vi "excavator1D_array.vi"(0 "Name":string, 1 "Array":dbl[][](array[numeric]) format="%#_13g", 2 "x_max":dbl, 3 "x_min":dbl, 4 "Save?":bool) -> (5 "xPoints":i32=263)   [LabVIEW 2013]
panel:
  in  "Tab Control":enum32{"Page 1", "Page 2"}(tab)
  in  "Ring":u16(ring)=1 items=["Windows", "Mac"]
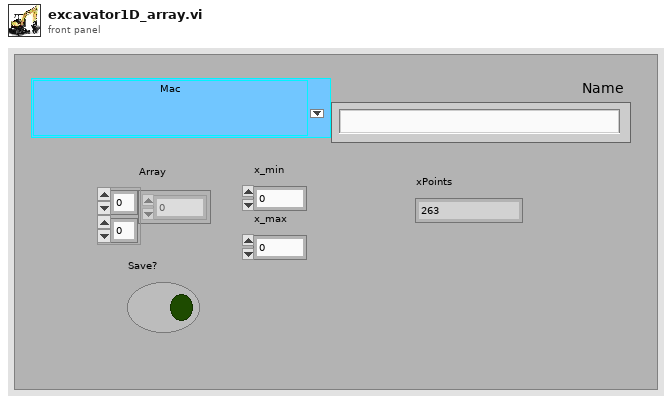
[diagram p1: front panel]
types:
  T1 = enum16{"open", "replace", "create", "open or create", "replace or create", "replace or create with confirmation"}
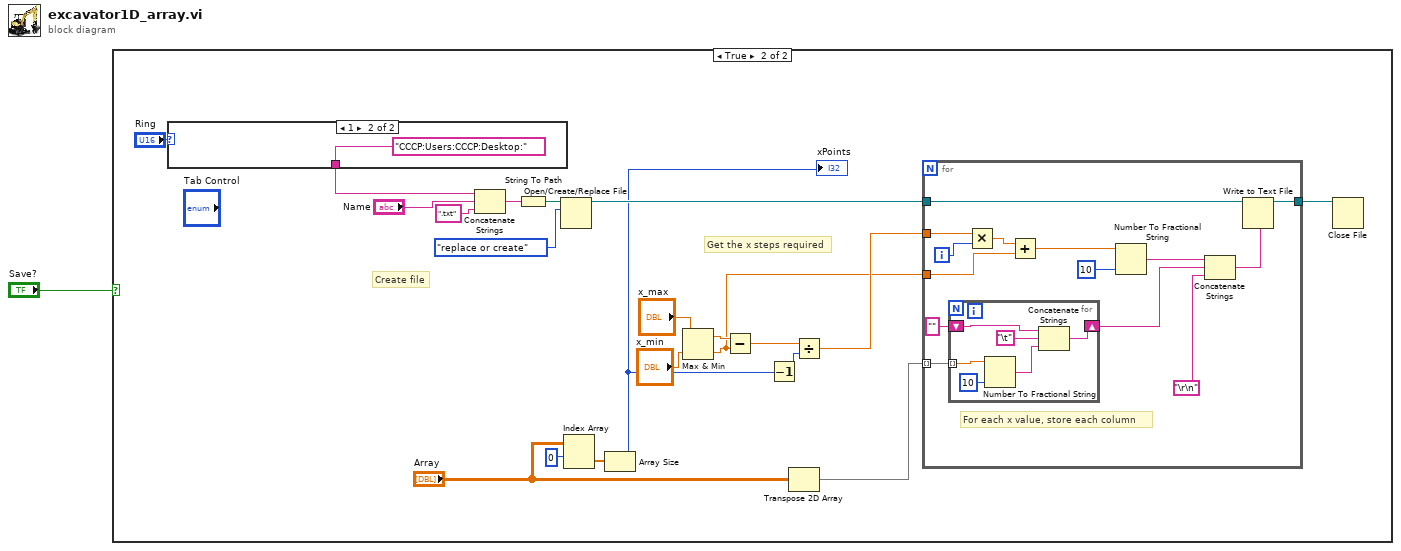
[diagram p0: block diagram]
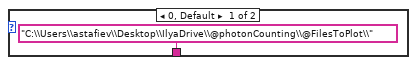
[diagram p3: hidden frame]
diagram:
  n1 = case shown="True" "Save?" {
    frame False {
    }
    frame True {
      # "Create file"
      # "Get the x steps required"
      n2 = case shown="1" "Ring" {
        tunnel: ["C:\\Users\\astafiev\\Desktop\\IlyaDrive\\@photonCounting\\@FilesToPlot\\" ("Directory") "CCCP:Users:CCCP:Desktop:" ("Directory")] -> w11
        frame 0, Default {
        }
        frame 1 {
        }
      }
      n3 = Concatenate Strings(w11, "Name", ".txt" ("FileName 2")) -> (w22:string)
      n4 = String To Path(string=w22) -> (path=w21:path)
      n5 = Open/Create/Replace File(file path (use dialog)=w21, operation (0:open)=T1."replace or create") -> (refnum out=w18:refnum<file>)  [unwired: 4 in, 2 out]
      n6 = Index Array(array="Array", index (row)=0) -> (element=w5:dbl[])  [unwired: 1 in]
      n7 = Array Size(array=w5) -> (size(s)=w9:i32)
      "xPoints" <- w9
      n8 = Max & Min(x="x_max", y="x_min") -> (max(x,y)=w14:dbl, min(x,y)=w13:dbl)
      n9 = Subtract(x=w14, y=w13) -> (x-y=w15:dbl)
      n10 = Decrement(x=w9) -> (x-1=w12:i32)
      n11 = Transpose 2D Array(2D array="Array") -> (transposed array=w2:dbl[][])
      n12 = Divide(x=w15, y=w12) -> (x/y=w16:dbl)
      n13 = for {
        tunnel: w18 -> [w36]
        tunnel: w16 -> [w35]
        tunnel: w13 -> [w32]
        tunnel: [w30] -> w4
        tunnel: w2 -> [w26] mode=indexing
        i -> [w34]
        # "For each x value, store each column"
        n14 = for {
          tunnel: w26 -> [w39] mode=indexing
          shift-right: [w42] -> w25
          shift-left: "" -> [w37]
          n15 = Number To Fractional String(number=w39, precision (6)=i16 10 ("width (-)")) -> (F-format string=w41:string)  [unwired: 2 in]
          n16 = Concatenate Strings(w37, "\t", w41) -> (w42:string)
        }
        n17 = Multiply(x=w35, y=w34) -> (x*y=w33:dbl)
        n18 = Add(x=w33, y=w32) -> (x+y=w31:dbl)
        n19 = Number To Fractional String(number=w31, precision (6)=i16 10 ("width (-)")) -> (F-format string=w29:string)  [unwired: 2 in]
        n20 = Concatenate Strings(w29, w25, "\r\n") -> (w28:string)
        n21 = Write to Text File(file (use dialog)=w36, text=w28) -> (refnum out=w30:refnum<file>)  [unwired: 2 in, 2 out]
      }
      n22 = Close File(refnum=w4) -> ()  [unwired: 1 in, 2 out]
    }
  }
